vi "ViperHawk Find Max Values.vi"(8 "Error In":errorcluster, 9 "Cycle Timer (Sec)":dbl format="%<%H:%M:%S>t", 10 "Cycle Stats":T1, 11 "Diagnostic Data Output":T2) -> (0 "Error Out":errorcluster, 3 "Cycle Stats Output":T1)   [LabVIEW 2016]
uses:
  Type Definitions/ViperHawk/ViperHawk Diagnostic Data.ctl
  Type Definitions/ViperHawk/ViperHawk Summary Stats.ctl
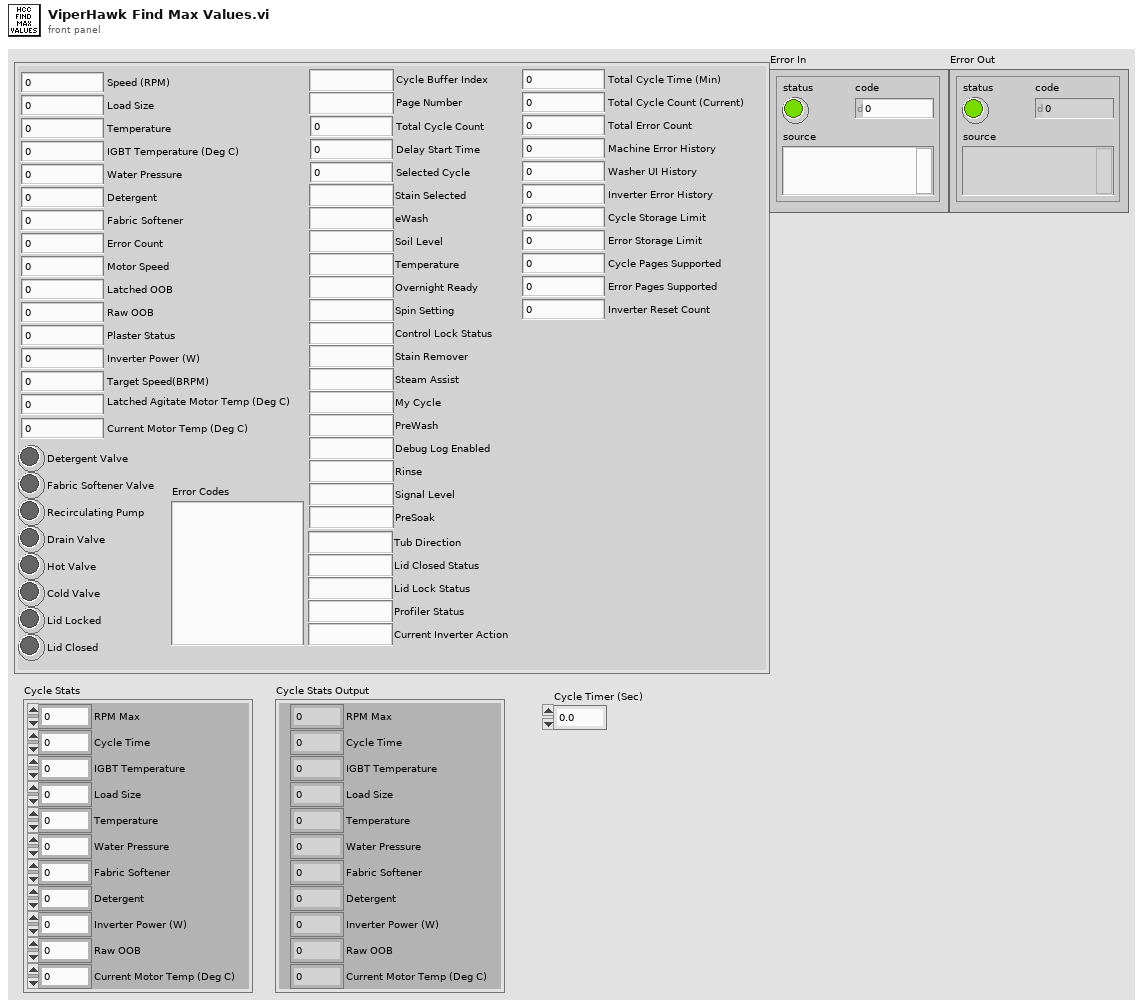
[diagram p1: front panel]
types:
  T1 = typedef "ViperHawk Summary Stats.ctl" = cluster{"RPM Max":u32, "Cycle Time":dbl, "IGBT Temperature":dbl, "Load Size":dbl, "Temperature":dbl, "Water Pressure":dbl, "Detergent":dbl, "Fabric Softener":dbl, "Inverter Power (W)":dbl, "Raw OOB":dbl, "Current Motor Temp (Deg C)":dbl}
  T2 = typedef "ViperHawk Diagnostic Data.ctl" = cluster{"Speed (RPM)":u32, "Load Size":u32, "Temperature":u32, "Water Pressure":dbl, "Detergent":u32, "Fabric Softener":u32, "Tub Direction":string, "Detergent Valve":bool, "Fabric Softener Valve":bool, "Recirculating Pump":bool, "Drain Valve":bool, "Hot Valve":bool, "Cold Valve":bool, "Lid Closed Status":string, "Lid Lock Status":string, "Error Count":u32, "IGBT Temperature (Deg C)":u32, "Motor Speed":u32, "Latched OOB":u32, "Raw OOB":u32, "Plaster Status":u32, "Inverter Power (W)":u32, "Target Speed(BRPM)":u32, "Latched Agitate Motor Temp (Deg C)":u32, "Current Motor Temp (Deg C)":u32, "Profiler Status":string, "Current Inverter Action":string, "Error Codes":string, "Lid Locked":bool, "Lid Closed":bool, "9E Diagnostic Data":cluster{"Total Cycle Time (Min)":u32, "Total Cycle Count (Current)":u16, "Total Error Count":u16, "Machine Error History":u32, "Washer UI History":u32, "Inverter Error History":u32, "Cycle Storage Limit":u8, "Error Storage Limit":u8, "Cycle Pages Supported":u8, "Error Pages Supported":u8, "Inverter Reset Count":u16}, "9F Diagnostic Data":cluster{"Cycle Buffer Index":string, "Page Number":string, "Total Cycle Count":u32, "Delay Start Time":u32, "Stain Selected":string, "Selected Cycle":u32, "eWash":string, "Soil Level":string, "Temperature":string, "Overnight Ready":string, "Spin Setting":string, "Control Lock Status":string, "Stain Remover":string, "Steam Assist":string, "My Cycle":string, "PreWash":string, "Debug Log Enabled":string, "Rinse":string, "Signal Level":string, "PreSoak":string}}
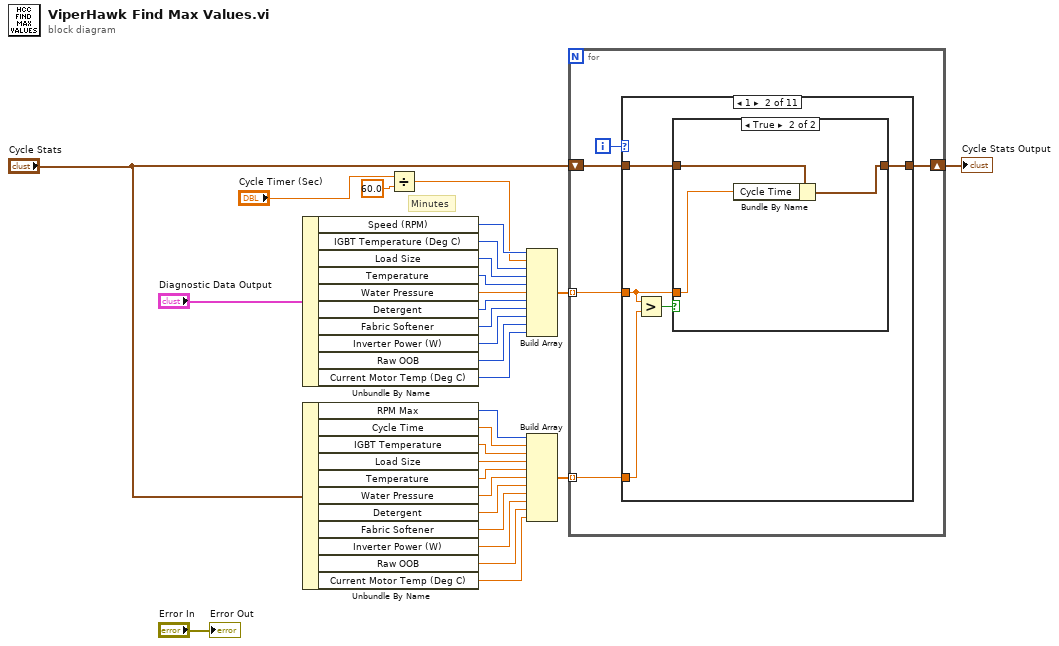
[diagram p0: block diagram]
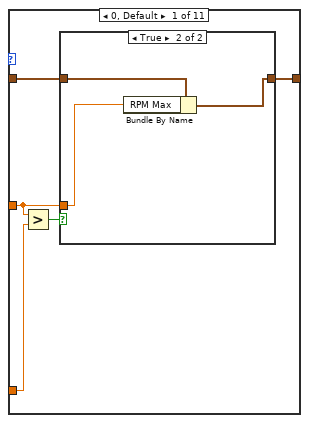
[diagram p2: hidden frame]
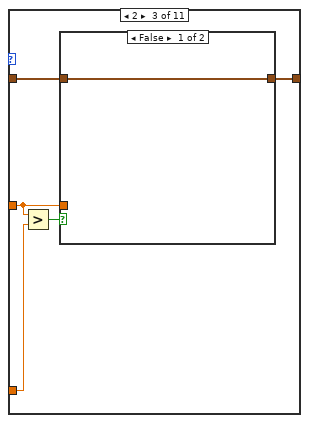
[diagram p5: hidden frame]
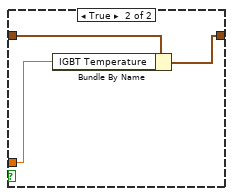
[diagram p6: hidden frame]
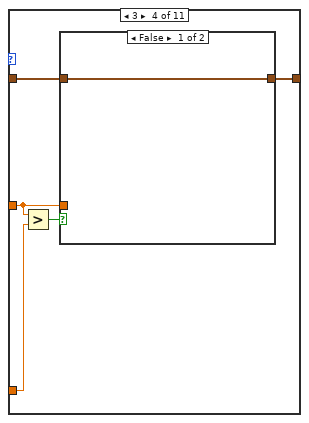
[diagram p7: hidden frame]
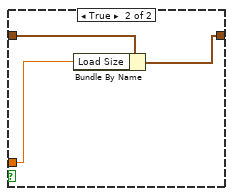
[diagram p8: hidden frame]
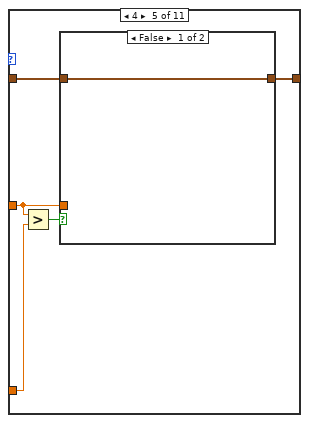
[diagram p9: hidden frame]
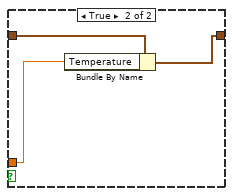
[diagram p10: hidden frame]
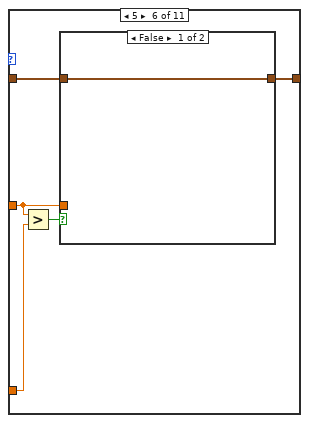
[diagram p11: hidden frame]
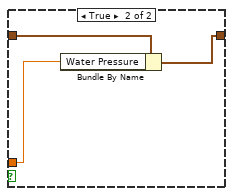
[diagram p12: hidden frame]
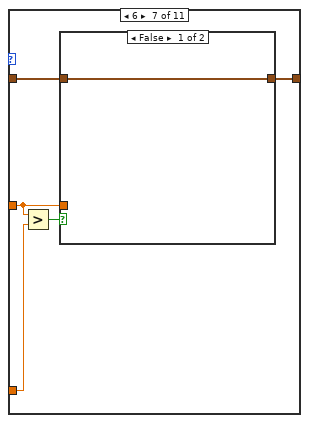
[diagram p13: hidden frame]
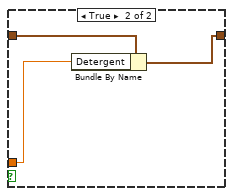
[diagram p14: hidden frame]
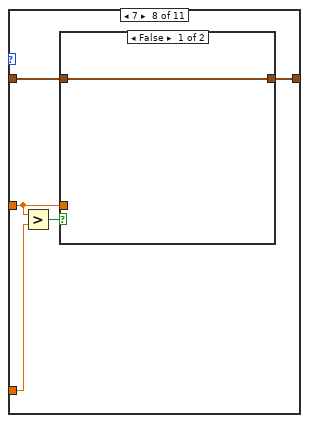
[diagram p15: hidden frame]
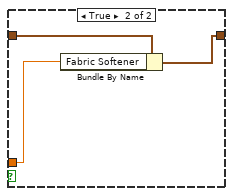
[diagram p16: hidden frame]
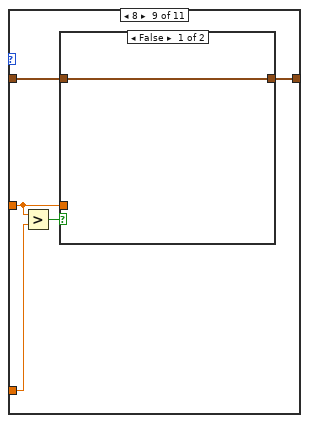
[diagram p17: hidden frame]
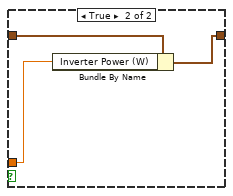
[diagram p18: hidden frame]
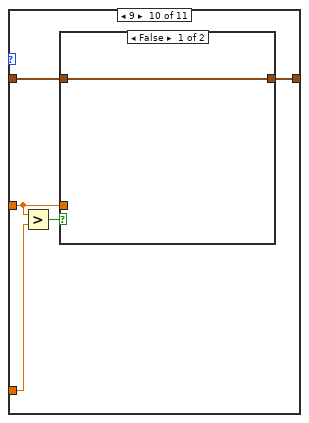
[diagram p19: hidden frame]
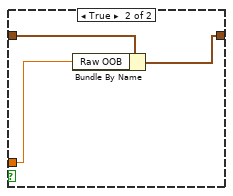
[diagram p20: hidden frame]
diagram:
  # "Minutes"
  n1 = Unbundle By Name("Diagnostic Data Output") -> ("Speed (RPM)"=w28:u32, "IGBT Temperature (Deg C)"=w27:u32, "Load Size"=w26:u32, "Temperature"=w25:u32, "Water Pressure"=w24:dbl, "Detergent"=w23:u32, "Fabric Softener"=w22:u32, "Inverter Power (W)"=w21:u32, "Raw OOB"=w20:u32, "Current Motor Temp (Deg C)"=w19:u32)
  n2 = Unbundle By Name("Cycle Stats") -> ("RPM Max"=w18:u32, "Cycle Time"=w17:dbl, "IGBT Temperature"=w16:dbl, "Load Size"=w15:dbl, "Temperature"=w14:dbl, "Water Pressure"=w13:dbl, "Detergent"=w12:dbl, "Fabric Softener"=w11:dbl, "Inverter Power (W)"=w10:dbl, "Raw OOB"=w9:dbl, "Current Motor Temp (Deg C)"=w8:dbl)
  n3 = Divide(x="Cycle Timer (Sec)", y=60.0) -> (x/y=w1:dbl)
  n4 = Build Array(w28, w1, w27, w26, w25, w24, w23, w22, w21, w20, w19) -> (w5:dbl[])
  n5 = Build Array(w18, w17, w16, w15, w14, w13, w12, w11, w10, w9, w8) -> (w4:dbl[])
  n6 = for {
    shift-right: [w33] -> w6
    shift-left: "Cycle Stats" -> [w34]
    tunnel: w5 -> [w32] mode=indexing
    tunnel: w4 -> [w31] mode=indexing
    i -> [w35]
    n7 = case shown="1" w35 {
      tunnel: w34 -> [w40 w49 w58 w67 w76 w85 w94 w103 w112 w121 w130]
      tunnel: [w39 w48 w57 w66 w75 w84 w93 w102 w111 w120 w129] -> w33
      tunnel: w32 -> [w36 w46 w54 w64 w73 w82 w91 w100 w109 w118 w127]
      tunnel: w31 -> [w38 w47 w55 w65 w74 w83 w92 w101 w110 w119 w128]
      frame 0, Default {
        n8 = Greater?(x=w36, y=w38) -> (0:w37:bool)
        n9 = case shown="True" w37 {
          tunnel: w40 -> [w41 w44]
          tunnel: [w41 w43] -> w39
          tunnel: w36 -> [_ w42]
          frame False {
          }
          frame True {
            n10 = Bundle By Name(cluster=w44, "RPM Max"=w42) -> (w43:T1)
          }
        }
      }
      frame 1 {
        n11 = Greater?(x=w46, y=w47) -> (0:w45:bool)
        n12 = case shown="True" w45 {
          tunnel: w49 -> [w50 w53]
          tunnel: [w50 w52] -> w48
          tunnel: w46 -> [_ w51]
          frame False {
          }
          frame True {
            n13 = Bundle By Name(cluster=w53, "Cycle Time"=w51) -> (w52:T1)
          }
        }
      }
      frame 2 {
        n14 = Greater?(x=w54, y=w55) -> (0:w56:bool)
        n15 = case shown="False" w56 {
          tunnel: w58 -> [w59 w62]
          tunnel: [w59 w61] -> w57
          tunnel: w54 -> [_ w60]
          frame False {
          }
          frame True {
            n16 = Bundle By Name(cluster=w62, "IGBT Temperature"=w60) -> (w61:T1)
          }
        }
      }
      frame 3 {
        n17 = Greater?(x=w64, y=w65) -> (0:w63:bool)
        n18 = case shown="False" w63 {
          tunnel: w67 -> [w68 w71]
          tunnel: [w68 w70] -> w66
          tunnel: w64 -> [_ w69]
          frame False {
          }
          frame True {
            n19 = Bundle By Name(cluster=w71, "Load Size"=w69) -> (w70:T1)
          }
        }
      }
      frame 4 {
        n20 = Greater?(x=w73, y=w74) -> (0:w72:bool)
        n21 = case shown="False" w72 {
          tunnel: w76 -> [w77 w80]
          tunnel: [w77 w79] -> w75
          tunnel: w73 -> [_ w78]
          frame False {
          }
          frame True {
            n22 = Bundle By Name(cluster=w80, "Temperature"=w78) -> (w79:T1)
          }
        }
      }
      frame 5 {
        n23 = Greater?(x=w82, y=w83) -> (0:w81:bool)
        n24 = case shown="False" w81 {
          tunnel: w85 -> [w86 w89]
          tunnel: [w86 w88] -> w84
          tunnel: w82 -> [_ w87]
          frame False {
          }
          frame True {
            n25 = Bundle By Name(cluster=w89, "Water Pressure"=w87) -> (w88:T1)
          }
        }
      }
      frame 6 {
        n26 = Greater?(x=w91, y=w92) -> (0:w90:bool)
        n27 = case shown="False" w90 {
          tunnel: w94 -> [w95 w98]
          tunnel: [w95 w97] -> w93
          tunnel: w91 -> [_ w96]
          frame False {
          }
          frame True {
            n28 = Bundle By Name(cluster=w98, "Detergent"=w96) -> (w97:T1)
          }
        }
      }
      frame 7 {
        n29 = Greater?(x=w100, y=w101) -> (0:w99:bool)
        n30 = case shown="False" w99 {
          tunnel: w103 -> [w104 w107]
          tunnel: [w104 w106] -> w102
          tunnel: w100 -> [_ w105]
          frame False {
          }
          frame True {
            n31 = Bundle By Name(cluster=w107, "Fabric Softener"=w105) -> (w106:T1)
          }
        }
      }
      frame 8 {
        n32 = Greater?(x=w109, y=w110) -> (0:w108:bool)
        n33 = case shown="False" w108 {
          tunnel: w112 -> [w113 w116]
          tunnel: [w113 w115] -> w111
          tunnel: w109 -> [_ w114]
          frame False {
          }
          frame True {
            n34 = Bundle By Name(cluster=w116, "Inverter Power (W)"=w114) -> (w115:T1)
          }
        }
      }
      frame 9 {
        n35 = Greater?(x=w118, y=w119) -> (0:w117:bool)
        n36 = case shown="False" w117 {
          tunnel: w121 -> [w122 w125]
          tunnel: [w122 w124] -> w120
          tunnel: w118 -> [_ w123]
          frame False {
          }
          frame True {
            n37 = Bundle By Name(cluster=w125, "Raw OOB"=w123) -> (w124:T1)
          }
        }
      }
      frame 10 {
        n38 = Greater?(x=w127, y=w128) -> (0:w126:bool)
        n39 = case shown="True" w126 {
          tunnel: w130 -> [w131 w134]
          tunnel: [w131 w133] -> w129
          tunnel: w127 -> [_ w132]
          frame False {
          }
          frame True {
            n40 = Bundle By Name(cluster=w134, "Current Motor Temp (Deg C)"=w132) -> (w133:T1)
          }
        }
      }
    }
  }
  "Cycle Stats Output" <- w6
  "Error Out" <- "Error In"
